vi "Update Number of Runners.vi"(8 "error in (no error)":errorcluster, 11 "Test Runner in":refnum<class "Test Runner.lvclass">) -> (0 "error out":errorcluster, 3 "Test Runner out":refnum<class "Test Runner.lvclass">)   [LabVIEW 2020, in "Test Runner.lvclass"]
uses:
  Test Runner.lvclass
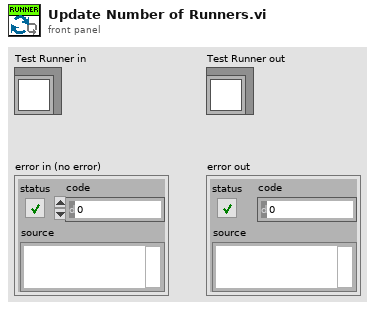
[diagram p1: front panel]
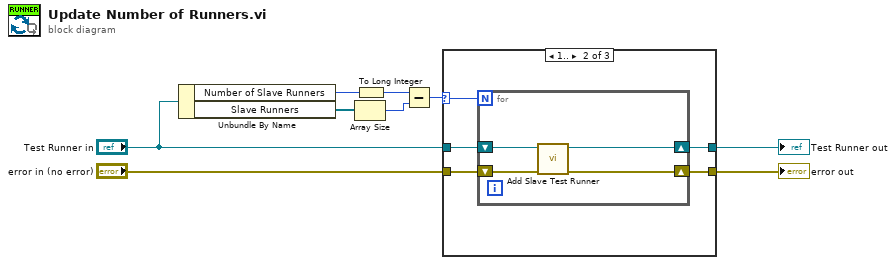
[diagram p0: block diagram]
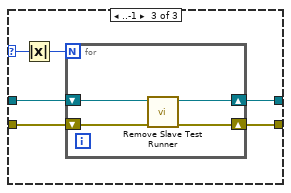
[diagram p3: hidden frame]
diagram:
  n1 = Unbundle By Name("Test Runner in") -> ("Number of Slave Runners"=w4:u32, "Slave Runners"=w5:refnum<class "Slave Test Runner.lvclass">[])
  n2 = Array Size(array=w5) -> (size(s)=w3:i32)
  n3 = To Long Integer(number=w4) -> (32bit integer=w1:i32)
  n4 = Subtract(x=w1, y=w3) -> (x-y=w2:i32)
  n5 = case shown="1.." w2 {
    selector: w2 -> [_ w12 w22]
    tunnel: [w11 w16 w26] -> w9
    tunnel: "Test Runner in" -> [w11 w15 w25]
    tunnel: "error in (no error)" -> [w10 w14 w24]
    tunnel: [w10 w13 w23] -> w6
    frame 0 {
    }
    frame 1.. {
      n6 = for {
        N: w12 -> [_]
        shift-right: [w20] -> w13
        shift-left: w14 -> [w19]
        shift-right: [w17] -> w16
        shift-left: w15 -> [w18]
        n7 = call "Add Slave Test Runner.vi"("error in (no error)"=w19, "Test Runner in"=w18) -> ("error out"=w20:errorcluster, "Test Runner out"=w17:refnum<class "Test Runner.lvclass">)  [unwired: 8 in]
      }
    }
    frame ..-1 {
      n8 = Absolute Value(x=w22) -> (abs(x)=w21:i32)
      n9 = for {
        N: w21 -> [_]
        shift-right: [w29] -> w23
        shift-left: w24 -> [w30]
        shift-right: [w27] -> w26
        shift-left: w25 -> [w28]
        n10 = call "Remove Slave Test Runner.vi"("error in (no error)"=w30, "Test Runner in"=w28) -> ("error out"=w29:errorcluster, "Test Runner out"=w27:refnum<class "Test Runner.lvclass">)  [unwired: 8 in]
      }
    }
  }
  "Test Runner out" <- w9
  "error out" <- w6
